vi "HXG2_ProgCntDowns.vi"(7 "FGVctrl":enum16{"Write", "Pass"}(ring), 8 "error in (no error)":errorcluster, 11 "Numeric":dbl) -> (0 "error out":errorcluster, 3 "Exec t (sec)":dbl)   [LabVIEW 2012]
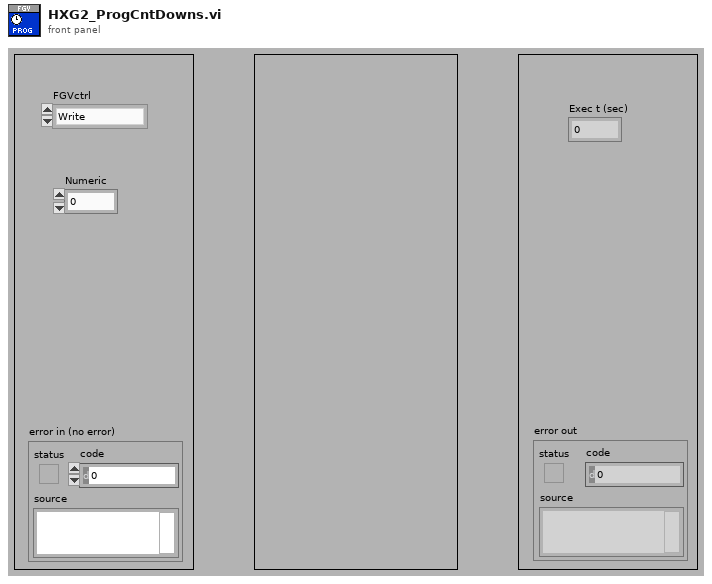
[diagram p1: front panel]
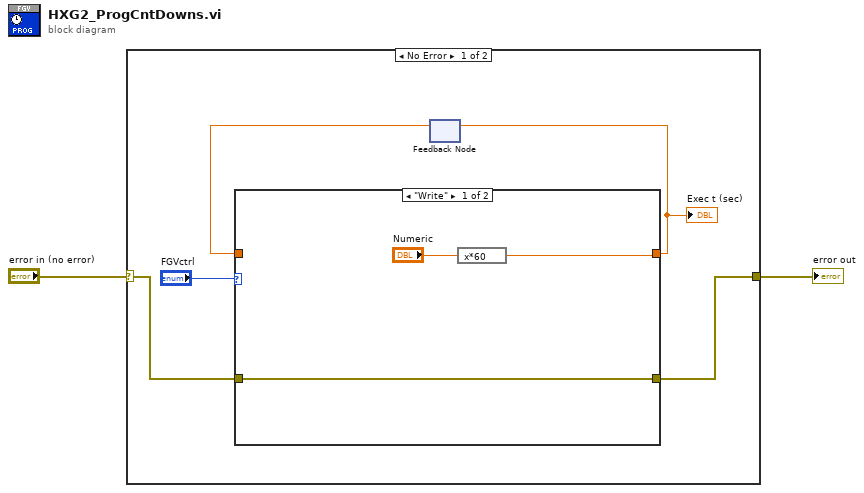
[diagram p0: block diagram]
diagram:
  n1 = case shown="No Error" "error in (no error)" {
    selector: "error in (no error)" -> [w4 w13]
    tunnel: [w3 w13] -> w2
    frame No Error {
      n2 = feedback #1() -> (w5:dbl)  [unwired: 1 in]
      n3 = case shown="\"Write\"" "FGVctrl" {
        tunnel: [w8 w12] -> w6
        tunnel: w5 -> [_ w12]
        tunnel: w4 -> [w9 w11]
        tunnel: [w9 w11] -> w3
        frame "Write" {
          n4 = expression code="x*60"("Numeric") -> (w8:dbl)
        }
        frame "Pass", Default {
        }
      }
      "Exec t (sec)" <- w6
      n5 = feedback-in #1(w6) -> ()
    }
    frame Error {
    }
  }
  "error out" <- w2
